vi "Correct Data.vi"(8 "error in (no error)":errorcluster, 10 "Data In":refnum<class "Data.lvclass">, 11 "PPT in":refnum<class "PPT.lvclass">) -> (0 "error out":errorcluster, 2 "Data Out":refnum<class "Data.lvclass">, 3 "PPT out":refnum<class "PPT.lvclass">)   [LabVIEW 2014, in "PPT Library.lvlib" / "PPT.lvclass"]
uses:
  PPT.lvclass
  reusable/Data/Data.lvclass
  Data/PPT Data.lvclass
  Configurable Device/Configurable Device.lvclass/Configurable Device.ctl
  Data/PPT Data.lvclass/PPT Data.ctl
  Data/Write P.vi
  Data/Read P.vi
  Configurable Device/Accessors/Read Cal Equation.vi
  <vilib>/gmath/NI_Gmath.lvlib
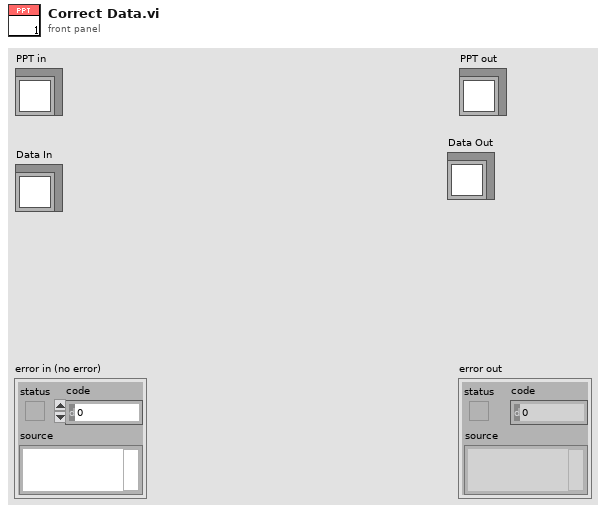
[diagram p1: front panel]
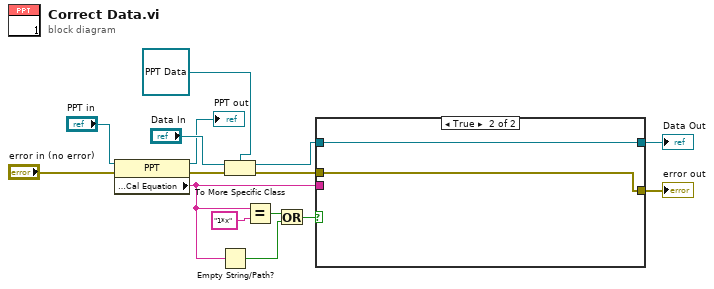
[diagram p0: block diagram]
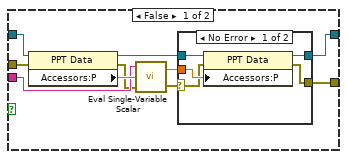
[diagram p2: hidden frame]
diagram:
  n1 = property class="PPT"(reference="PPT in", error in="error in (no error)") -> (reference out=→"PPT out":refnum<class "PPT.lvclass">, error out=w3:errorcluster, "Accessors:Cal Equation"=w7:string)
  n2 = Empty String/Path?(string/path=w7) -> (empty?=w9:bool)
  n3 = To More Specific Class(target class=refnum<class "PPT Data.lvclass"> refnum ("PPT Library.lvlib:PPT Data"), reference="Data In", error in=w3) -> (specific class reference=w12:refnum<class "PPT Data.lvclass">, error out=w2:errorcluster)
  n4 = Equal?(x=w7, y="1*x") -> (x = y?=w10:bool)
  n5 = Or(x=w10, y=w9) -> (x .or. y?=w8:bool)
  n6 = case shown="True" w8 {
    tunnel: w12 -> [w25 w33]
    tunnel: w7 -> [w23 _]
    tunnel: [w19 w33] -> w6
    tunnel: [w18 w32] -> w1
    tunnel: w2 -> [w16 w32]
    frame False {
      n7 = property class="PPT Data"(reference=w25, error in=w16) -> (reference out=w22:refnum<class "PPT Data.lvclass">, error out=w17:errorcluster, "Accessors:P"=w24:dbl)
      n8 = call <vilib>:"Eval Single-Variable Scalar.vi"("error in (no error)"=w17, "x value"=w24, "formula"=w23) -> ("error out"=w21:errorcluster, "y value"=w20:dbl)
      n9 = case shown="No Error" w21 {
        selector: w21 -> [w27 _]
        tunnel: w22 -> [w30 w31]
        tunnel: w20 -> [w29 _]
        tunnel: [w28 w31] -> w19
        tunnel: [w26 _] -> w18
        frame No Error {
          n10 = property class="PPT Data"(reference=w30, error in=w27, "Accessors:P"=w29) -> (reference out=w28:refnum<class "PPT Data.lvclass">, error out=w26:errorcluster)
        }
        frame Error {
        }
      }
    }
    frame True {
    }
  }
  "error out" <- w1
  "Data Out" <- w6
